vi "Destroy Local Instance Events.vi"(8 "error in":errorcluster, 11 "Module ID":i32) -> (0 "error out":errorcluster)   [LabVIEW 2019, in "Inversor.lvlib"]
doc: "_____\nCreated using DQMH Framework: Event Scripter 7.1.0.1503."
uses:
  Inversor.lvlib
  Local Instance Events SEQ/Local Instance Events SEQ.lvlib
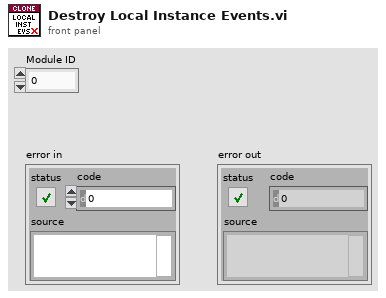
[diagram p1: front panel]
types:
  T1 = typedef "Inversor.lvlib/Request Events--cluster.ctl" = cluster{"Stop Module":refnum<user-event>, "Show Panel":refnum<user-event>, "Hide Panel":refnum<user-event>, "Show Diagram":refnum<user-event>, "Get Module Execution Status":refnum<user-event>, "Local Instance":T2, "Private.Request Privado":refnum<user-event>, "Set Voltage":refnum<user-event>, "Request Simple":refnum<user-event>}
  T2 = typedef "Inversor.lvlib/Local Instance Request Events--cluster.ctl" = cluster{"Request Privado Local":refnum<user-event>}
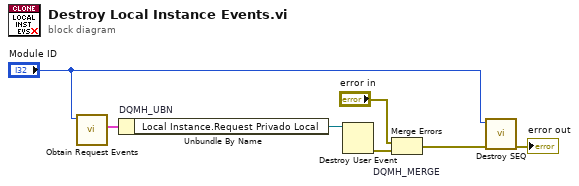
[diagram p0: block diagram]
diagram:
  n1 = call "Obtain Request Events.vi"("Module ID"="Module ID") -> ("Inversor Request Events"=w4:T1)  [unwired: 9 in, 1 out]
  n2 = Unbundle By Name "DQMH_UBN"(w4) -> ("Local Instance.Request Privado Local"=w6:refnum<user-event>)
  n3 = Destroy User Event(user event=w6) -> (error out=w5:errorcluster)  [unwired: 1 in]
  n4 = Merge Errors "DQMH_MERGE"("error in", w5) -> (w3:errorcluster)
  n5 = call "Destroy SEQ.vi"("error in"=w3, "Module ID"="Module ID") -> ("error out"=→"error out":errorcluster)  [unwired: 9 in]
